vi "String Array to Text File.vi"(1 "Array":string[](array[string]), 2 "file (use dialog)":path) -> ()   [LabVIEW 2014]
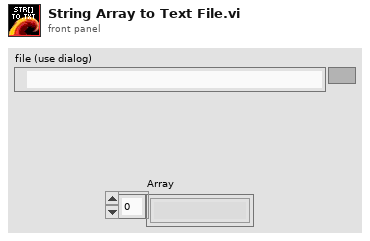
[diagram p1: front panel]
types:
  T1 = enum16{"open", "replace", "create", "open or create", "replace or create", "replace or create with confirmation"}
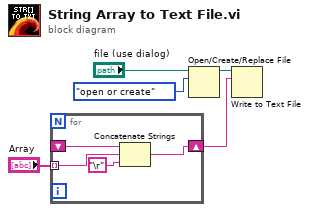
[diagram p0: block diagram]
diagram:
  n1 = for {
    tunnel: "Array" -> [w6] mode=indexing
    shift-right: [w8] -> w4
    shift-left: _ -> [w7]
    n2 = Concatenate Strings(w7, w6, "\r") -> (w8:string)
  }
  n3 = Open/Create/Replace File(file path (use dialog)="file (use dialog)", operation (0:open)=T1."open or create") -> (refnum out=w1:refnum<file>)  [unwired: 4 in, 2 out]
  n4 = Write to Text File(file (use dialog)=w1, text=w4) -> ()  [unwired: 2 in, 3 out]
